vi "Master GUI Template.vi"() -> ()   [LabVIEW 2020]
uses:
  tcp_new_data_event.ctl
  tcp new data cluster.ctl
panel:
  out "error IO 2":errorcluster
  out "tcp data event":T1
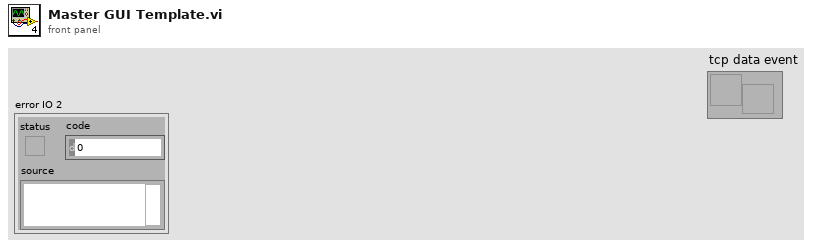
[diagram p1: front panel]
types:
  T1 = typedef "tcp_new_data_event.ctl" = refnum<user-event>
  T2 = typedef "tcp new data cluster.ctl" = cluster{"EventEnum":enum16{"new data", "connection status update"}, "Device name":string}
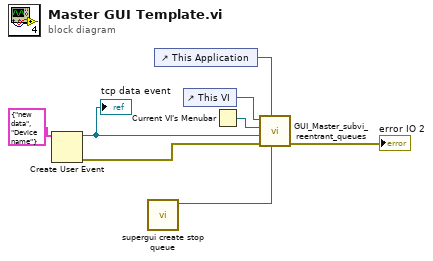
[diagram p0: block diagram]
diagram:
  n1 = Create User Event(user event datatype=T2 {"EventEnum"=enum."new data", "Device name"="Device name"} ("New Event")) -> (user event=w8:refnum<user-event>, error out=w4:errorcluster)  [unwired: 1 in]
  "tcp data event" <- w8
  n2 = call "supergui create stop queue.vi"() -> ("STOP Queue out"=w1:refnum<queue>)  [unwired: 11 in]
  n3 = control-ref of="This Application"() -> (w3:refnum<vi>)
  n4 = control-ref of="This VI"() -> (w7:refnum<vi>)
  n5 = Current VI's Menubar() -> (w6:refnum<k9>)
  n6 = call "GUI_Master_subvi_reentrant_queues.vi"("STOP Queue in"=w1, "This Application"=w3, "error in (no error)"=w4, "tcp data event"=w8, "Caller menu reference"=w6, "Caller VI ref"=w7) -> ("error out"=→"error IO 2":errorcluster)  [unwired: 5 in]
